vi "Q8381 Disp Wave Data Graph.vi"(4 "Filename:":path=path "C:/Users/H-Lab/Desktop/test.lvm" caption="Filename", 5 "Log/Lin Scale":u16(ring) items=["LOG Scale", "LINEAR Scale"], 6 "Take Spectra":bool, 7 "SpanFull":bool, 8 "Stop Program":bool, 9 "Refresh Graph":bool, 10 "VISA resource name":refnum<visa-resource-name>, 11 "GPIB address":u16=8 step=1) -> (0 "center":dbl format="%#.5f", 1 "GPIB status":bool, 2 "UNCAL":bool, 3 "OSA Graph":T1(graph))   [LabVIEW 2017]
panel:
  in  "Comment for Data Set":string caption="Comment"
  out "Y unit":string
  in  "(LOG SCALE ONLY)":u16(ring) items=["10dB/D", "5dB/D", "2dB/D", "1dB/D", "0.5dB/D", "0.2dB/D"]
  in  "Line or Log":bool
  in  "Save data":bool
  in  "Ref Level Peak":bool
  in  "Center":bool
  in  "Options 2":u16(ring) items=["Stop", "Single", "Repeat"]
  in  "Options":u16(ring) items=["0.1nm", "0.2nm", "0.5nm", "1.0nm", "2.0nm", "5.01nm"]
  in  "Resolution":bool
  in  "Ref Level\nAuto":bool
  in  "unit/off/on":u16(ring) items=["dBm", "mW", "uW", "nW"]
  in  "Set Ref Value":dbl format="%#.6f"
  in  "Ref Level\nSet":bool
  in  "SpanStop":bool
  in  "unit/off/on":u16(ring) items=["um ", "nm"]
  in  "Set Stop Value":dbl format="%#.6f"
  in  "unit/off/on":u16(ring) items=["um ", "nm"]
  in  "Set Start Value":dbl format="%#.6f"
  in  "SpanStart":bool
  in  "unit/off/on":u16(ring) items=["um ", "nm"]
  in  "Set value":dbl format="%#.6f"
  in  "Func":u16(ring) items=["CENTER", "PEAK", "CURSOR"]
  # "FUNCTION"
  # "AND"
  # "OR"
  # "um"
  # "CenterValue:"
  # "To save the file in  Microsoft Excel, remove \".lvm\" \nand manually input the file extension \".csv\"."
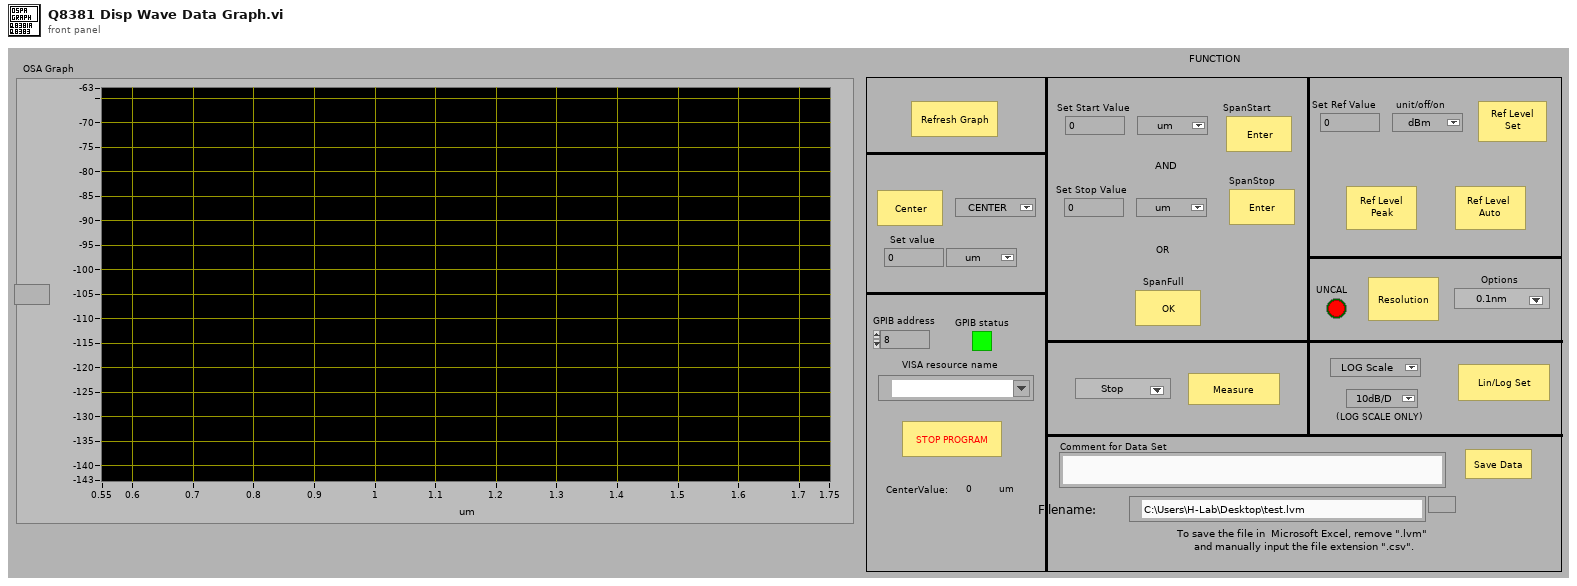
[diagram p1: front panel]
types:
  T1 = cluster{"X Axis Data":dbl[], "Y Axis Data":dbl[]}
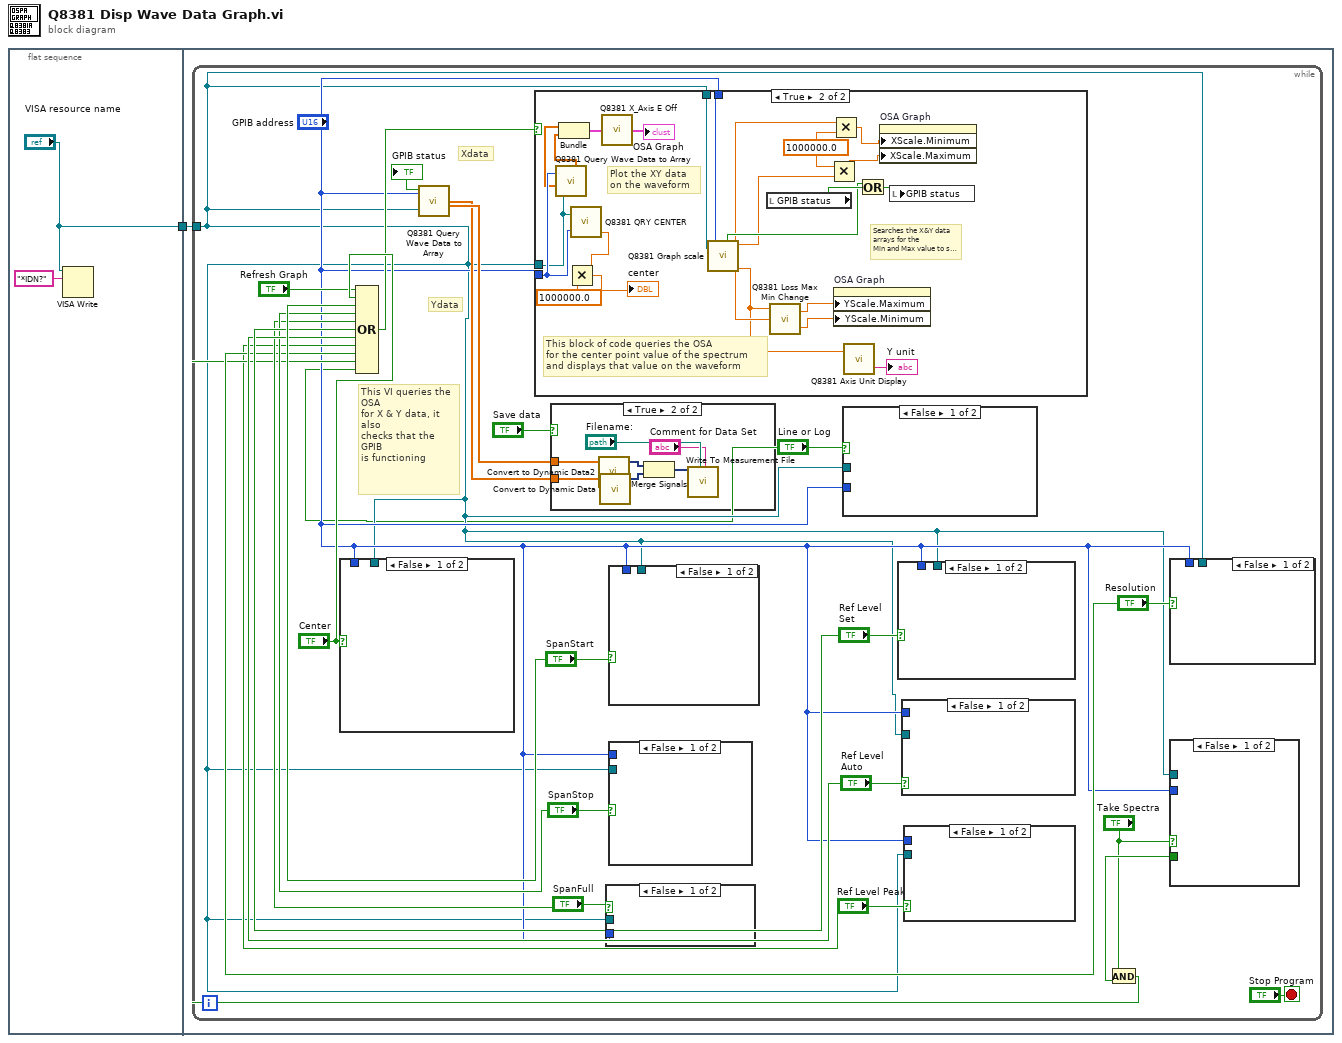
[diagram p0: block diagram]
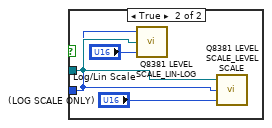
[diagram p2: hidden frame]
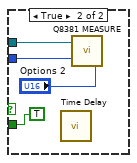
[diagram p5: hidden frame]
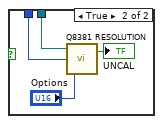
[diagram p6: hidden frame]
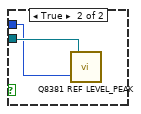
[diagram p7: hidden frame]
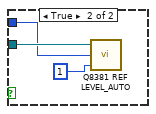
[diagram p8: hidden frame]
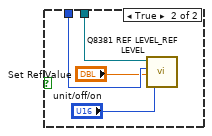
[diagram p9: hidden frame]
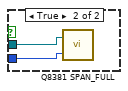
[diagram p10: hidden frame]
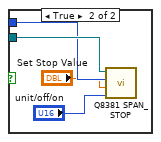
[diagram p11: hidden frame]
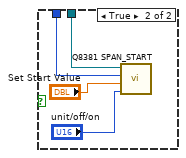
[diagram p12: hidden frame]
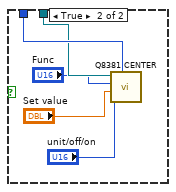
[diagram p13: hidden frame]
diagram:
  n1 = flat-sequence {
    tunnel: ["VISA resource name"] -> w1
    tunnel: w1 -> [w4]
    frame #0 {
      n2 = VISA Write(VISA resource name="VISA resource name", write buffer="*IDN?") -> ()  [unwired: 1 in, 3 out]
    }
    frame #1 {
      n3 = while {
        tunnel: w4 -> [w7]
        stop <- "Stop Program" stop-if-true
        # "Ydata"
        # "Xdata"
        # "This VI queries the OSA\nfor X & Y data, it also\nchecks that the GPIB\nis functioning"
        n4 = case shown="False" "Center" {
          tunnel: "GPIB address" -> [_ w92]
          tunnel: w7 -> [_ w91]
          frame False {
          }
          frame True {
            n5 = call "Q8381 CENTER.vi"("VISA resource name"=w91, "Func"="Func", "Set value"="Set value", "unit/off/on"="unit/off/on", "GPIB Address"=w92) -> ()  [unwired: 1 out]
          }
        }
        n6 = call "Q8381 Query Wave Data to Array.vi"("VISA resource name"=w7, "GPIB address"="GPIB address") -> ("X Axis Data"=w10:dbl[], "GPIB status"=→"GPIB status":bool, "Y Axis Data"=w9:dbl[])  [unwired: 1 in, 1 out]
        n7 = case shown="True" "Save data" {
          tunnel: w10 -> [_ w33]
          tunnel: w9 -> [_ w32]
          frame False {
          }
          frame True {
            n8 = call "Convert to Dynamic Data2"("Array"=w33) -> ("Dynamic Data Type"=w36:dynamicdata)  [unwired: 3 in]
            n9 = call "Convert to Dynamic Data"("Array"=w32) -> ("Dynamic Data Type"=w34:dynamicdata)  [unwired: 3 in]
            n10 = Merge Signals(w36, w34) -> (w35:dynamicdata)
            n11 = call "Write To Measurement File"("Signals"=w35, "Filename"="Filename:", "Comment"="Comment for Data Set") -> ()  [unwired: 14 in, 3 out]
          }
        }
        n12 = case shown="False" "SpanFull" {
          tunnel: "GPIB address" -> [_ w78]
          tunnel: w7 -> [_ w79]
          frame False {
          }
          frame True {
            n13 = call "Q8381 SPAN_FULL.vi"("GPIB Address"=w78, "VISA resource name"=w79) -> ()  [unwired: 1 out]
          }
        }
        n14 = case shown="False" "SpanStart" {
          tunnel: "GPIB address" -> [_ w86]
          tunnel: w7 -> [_ w87]
          frame False {
          }
          frame True {
            n15 = call "Q8381 SPAN_START.vi"("unit"="unit/off/on", "value"="Set Start Value", "GPIB Address"=w86, "VISA resource name"=w87) -> ()  [unwired: 1 out]
          }
        }
        n16 = case shown="False" "SpanStop" {
          tunnel: "GPIB address" -> [_ w81]
          tunnel: w7 -> [_ w82]
          frame False {
          }
          frame True {
            n17 = call "Q8381 SPAN_STOP.vi"("unit"="unit/off/on", "value"="Set Stop Value", "GPIB Address"=w81, "VISA resource name"=w82) -> ()  [unwired: 1 out]
          }
        }
        n18 = case shown="False" "Line or Log" {
          tunnel: "GPIB address" -> [_ w26]
          tunnel: w7 -> [_ w27]
          frame False {
          }
          frame True {
            n19 = call "Q8381 LEVEL SCALE_LIN-LOG.vi"("off/on"="Log/Lin Scale", "VISA resource name"=w27, "GPIB Address"=w26) -> ()  [unwired: 1 out]
            n20 = call "Q8381 LEVEL SCALE_LEVEL SCALE.vi"("scale"="(LOG SCALE ONLY)", "GPIB Address"=w26, "VISA resource name"=w27) -> ()  [unwired: 1 out]
          }
        }
        n21 = case shown="False" "Ref Level\nSet" {
          tunnel: "GPIB address" -> [_ w76]
          tunnel: w7 -> [_ w77]
          frame False {
          }
          frame True {
            n22 = call "Q8381 REF LEVEL_REF LEVEL.vi"("unit"="unit/off/on", "value"="Set Ref Value", "GPIB Address"=w76, "VISA resource name"=w77) -> ()  [unwired: 1 out]
          }
        }
        n23 = case shown="False" "Ref Level\nAuto" {
          tunnel: "GPIB address" -> [_ w72]
          tunnel: w7 -> [_ w73]
          frame False {
          }
          frame True {
            n24 = call "Q8381 REF LEVEL_AUTO.vi"("off/on"=1, "GPIB Sddress"=w72, "VISA resource name"=w73) -> ()  [unwired: 1 out]
          }
        }
        n25 = case shown="False" "Ref Level Peak" {
          tunnel: "GPIB address" -> [_ w69]
          tunnel: w7 -> [_ w70]
          frame False {
          }
          frame True {
            n26 = call "Q8381 REF LEVEL_PEAK.vi"("GPIB Address"=w69, "VISA resource name"=w70) -> ()  [unwired: 1 out]
          }
        }
        n27 = case shown="False" "Resolution" {
          tunnel: "GPIB address" -> [_ w67]
          tunnel: w7 -> [_ w68]
          frame False {
          }
          frame True {
            n28 = call "Q8381 RESOLUTION.vi"("resolution"="Options", "GPIB Address"=w67, "VISA resource name"=w68) -> ("UNCAL"=→"UNCAL":bool)  [unwired: 1 out]
          }
        }
        n29 = case shown="False" "Take Spectra" {
          tunnel: "GPIB address" -> [_ w62]
          tunnel: [_ TRUE] -> w17
          tunnel: w7 -> [_ w63]
          frame False {
          }
          frame True {
            n30 = call "Time Delay"() -> ()  [unwired: 11 in, 1 out]
            n31 = call "Q8381 MEASURE.vi"("Meas mode"="Options 2", "GPIB Address"=w62, "VISA resource name"=w63) -> ()  [unwired: 1 out]
          }
        }
        n32 = And(x="Take Spectra", y=w17) -> (x .and. y?=w18:bool)
        n33 = Compound Arithmetic op=OR("Refresh Graph", "Center", "SpanStart", "SpanStop", "SpanFull", "Ref Level\nSet", "Ref Level\nAuto", "Ref Level Peak", "Resolution", w18, "Line or Log") -> (w12:bool)
        n34 = case shown="True" w12 {
          tunnel: w7 -> [_ w47]
          tunnel: "GPIB address" -> [_ w46]
          tunnel: w7 -> [_ w42]
          tunnel: "GPIB address" -> [_ w43]
          frame False {
          }
          frame True {
            w60 = 1000000.0
            # "Searches the X&Y data arrays for the\nMin and Max value to set the scale \nof the waveform graph."
            # "This block of code queries the OSA \nfor the center point value of the spectrum\nand displays that value on the waveform"
            # "Plot the XY data \non the waveform"
            n35 = call "Q8381 Query Wave Data to Array.vi"("VISA resource name"=w42, "GPIB address"=w43) -> ("X Axis Data"=w40:dbl[], "Y Axis Data"=w41:dbl[])  [unwired: 1 in, 2 out]
            n36 = Bundle("X Axis Data"=w40, "Y Axis Data"=w41) -> (w39:T1)  [unwired: 1 in]
            n37 = call "Q8381 QRY CENTER.vi"("VISA resource name"=w42, "GPIB Address"=w43) -> ("Center value"=w51:dbl)  [unwired: 2 out]
            n38 = Multiply(x=w51, y=1000000.0) -> (x*y=→"center":dbl)
            n39 = call "Q8381 X_Axis E Off.vi"("Graph Data"=w39) -> ("Out Data"=→"OSA Graph":T1)
            n40 = call "Q8381 Graph scale.vi"("GPIB Address"=w46, "VISA resource name"=w47) -> ("Y max"=w45:dbl, "Y min"=w55:dbl, "X min"=w53:dbl, "X max"=w52:dbl, "GPIB Status"=w54:bool)
            n41 = local read "GPIB status"() -> (w57:bool)
            n42 = call "Q8381 Loss Max Min Change .vi"("Received Y: min"=w55, "Received Y: max"=w45) -> ("Y: min"=w37:dbl, "Y: max"=w38:dbl)  [unwired: 1 in]
            n43 = Multiply(x=w60, y=w52) -> (x*y=w48:dbl)
            n44 = Multiply(x=w53, y=w60) -> (x*y=w49:dbl)
            n45 = property on="OSA Graph" class="XYGraph (strict)"("YScale.Maximum"=w38, "YScale.Minimum"=w37) -> ()  [unwired: 2 in, 2 out]
            n46 = call "Q8381 Axis Unit Display.vi"("Y Input"=w45) -> ("Y unit"=→"Y unit":string)  [unwired: 1 in, 1 out]
            n47 = Or(x=w54, y=w57) -> (x .or. y?=w58:bool)
            n48 = property on="OSA Graph" class="XYGraph (strict)"("XScale.Minimum"=w49, "XScale.Maximum"=w48) -> ()  [unwired: 2 in, 2 out]
            n49 = local write "GPIB status"(w58) -> ()
          }
        }
      }
    }
  }
